vi "Append Bolded Text to Report.vi"(4 "MS Office parameters":T1, 5 "error in":errorcluster, 6 "On new line?":bool, 7 "Text":string, 8 "report in":refnum<class "NI_report.lvclass">) -> (0 "error out":errorcluster, 1 "end out (Word)":i32, 2 "start out (Word)":i32, 3 "report out":refnum<class "NI_report.lvclass">)   [LabVIEW 2020, in "NI_ReportGenerationCore.lvlib"]
uses:
  <vilib>/Utility/NIReport.llb/NI_ReportGenerationCore.lvlib
  <vilib>/Utility/NIReport.llb/NI_report.lvclass
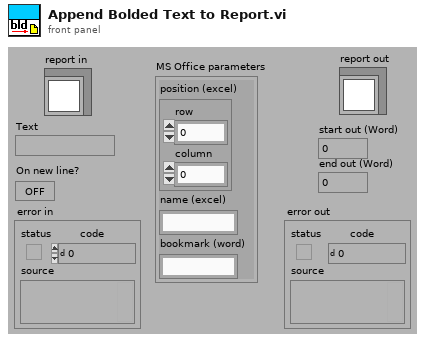
[diagram p1: front panel]
types:
  T1 = cluster{"position (excel)":cluster{"row":i32, "column":i32}, "name (excel)":string, "bookmark (word)":string}
  T2 = cluster{"Italic":enum16{"Italic Unchanged", "Italic On", "Italic Off"}, "Strike Through":enum16{"Strike Through Unchanged", "Strike Through On", "Strike Through Off"}, "Underline":enum16{"Underline Unchanged", "Underline On", "Underline Off"}, "Bold":enum16{"Bold Unchanged", "Bold On", "Bold Off"}}
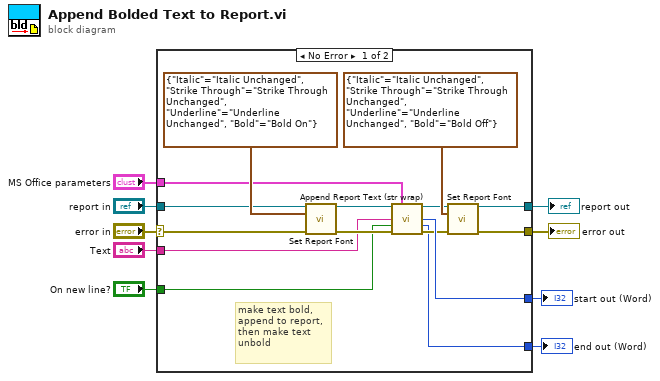
[diagram p0: block diagram]
diagram:
  n1 = case shown="No Error" "error in" {
    selector: "error in" -> [w19 w25]
    tunnel: [w23 w25] -> w9
    tunnel: [w22 w26] -> w8
    tunnel: "report in" -> [w20 w26]
    tunnel: "Text" -> [w15 _]
    tunnel: "On new line?" -> [w14 _]
    tunnel: "MS Office parameters" -> [w13 _]
    tunnel: [w10 _] -> w1
    tunnel: [w12 _] -> w2
    frame No Error {
      # "make text bold,\nappend to report,\nthen make text\nunbold"
      n2 = call-dynamic "Set Report Font.vi"("report in"=w20, "text options"=T2 {"Italic"=enum."Italic Unchanged", "Strike Through"=enum."Strike Through Unchanged", "Underline"=enum."Underline Unchanged", "Bold"=enum."Bold On"}, "error in (no error)"=w19) -> ("report out"=w17:refnum<class "NI_report.lvclass">, "error out"=w18:errorcluster)  [unwired: 10 in, 1 out]
      n3 = call <vilib>:"Append Report Text (str wrap).vi"("report in"=w17, "MS Office parameters"=w13, "text"=w15, "append on new line? (F)"=w14, "error in (no error)"=w18) -> ("report out"=w16:refnum<class "NI_report.lvclass">, "start out (Word)"=w12:i32, "end out (Word)"=w10:i32, "error out"=w11:errorcluster)  [unwired: 7 in]
      n4 = call-dynamic "Set Report Font.vi"("report in"=w16, "text options"=T2 {"Italic"=enum."Italic Unchanged", "Strike Through"=enum."Strike Through Unchanged", "Underline"=enum."Underline Unchanged", "Bold"=enum."Bold Off"}, "error in (no error)"=w11) -> ("report out"=w22:refnum<class "NI_report.lvclass">, "error out"=w23:errorcluster)  [unwired: 10 in, 1 out]
    }
    frame Error {
    }
  }
  "error out" <- w9
  "report out" <- w8
  "start out (Word)" <- w2
  "end out (Word)" <- w1
